vi "DependencyViewer_OnPopupMenu.vi"(11 "Object":u64) -> ()   [LabVIEW 2020]
uses:
  DependencyViewer/DependencyViewer.lvlib
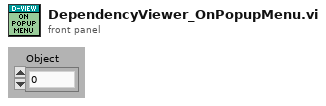
[diagram p1: front panel]
types:
  T1 = typedef "mxLvMenuItem.ctl" = cluster{"Menu Name":string, "Description":string, "Icon File Name":path, "Menu Tag":string, "Enabled":bool, "Checked":bool, "Separator":bool, "Batchable":bool, "Weight":i32, "Batch Mode (Ignored if Not Batchable)":enum32{"Show If All Items Support Command", "Show If Any Items Support Command"}, "Menu Location":enum32{"<None>", "Project", "Project / Build Specifications", "Tools", "Tools / Source Control", "Tools / Real-Time Module", "Help"}, "Exclude From Getting Started Window Menu":bool}
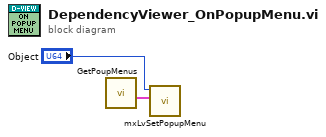
[diagram p0: block diagram]
diagram:
  n1 = call "GetPoupMenus.vi"() -> ("PopUpMenu(IfExists)"=w1:T1[])  [unwired: 11 in]
  n2 = call <resource>:"mxLvSetPopupMenu.vi"("Popup Menu Items"=w1, "Item"="Object") -> ()  [unwired: 8 in, 2 out]
